vi "Physical Learning v2.vi"(4 "Learning Gains":dbl[](array[numeric])=[1.0, 1.0, 1.0, 0.0], 6 "PID Cluster":T4={"L1 to L4 PID Cluster"={"L1 PID Gains"={"Kp"=0.005, "Kd"=0.5, "Ki"=0.0005}, "L2 PID Gains"={"Kp"=0.01, "Kd"=1.0, "Ki"=0.005}, "L3 PID Gains"={"Kp"=0.05, "Kd"=1.0, "Ki"=0.0005}, "L4 PID Gains"={"Kp"=0.1, "Kd"=0.1, "Ki"=0.0005}}, "Stage PID Cluster"={"Stage Z PID"={"Kp"=0.0005, "Kd"=0.001, "Ki"=0.0}, "Stage Y PID"={"Kp"=0.0003, "Kd"=0.01, "Ki"=0.0}, "Stage X PID"={"Kp"=0.0003, "Kd"=0.01, "Ki"=0.0}}, "OCT Z PID Gains"={"Kp"=0.0003, "Kd"=0.0001, "Ki"=0.01}}, 7 "Input RUY":T5, 8 "error in":errorcluster, 9 "Offset Home 2 RCM":dbl[](array[numeric])=[0.0, 0.0, 0.0, 0.0], 10 "Prev Posit Cluster":T3={"Prev L1 to L4 Posit"=[-0.5319, -0.035669172703475985, -2.0566170657346783, 0.9099264705882353], "Prev Stage Posit"=[6.002553885707208, 5.996566124542428, 5.995469940427586], "Prev OCT Z Posit"=-0.0}, 11 "FPGA VI Reference In":refnum<k20>) -> (0 "error out":errorcluster, 1 "Updated Trajectory":T1, 2 "Last Posit Cluster":T2={"Last L1 to L4 Posit"=[0.0, 0.0, 0.0, 0.0], "Last Stage Posit"=[6.0, 6.0, 6.0], "Last OCT Z Posit"=0.0}, 3 "FPGA VI Reference Out":refnum<k20>, 5 "Updated RUY":T5)   [LabVIEW 2016]
uses:
  <vilib>/Platform/TimedLoop/XDataNode/timing_clust.ctl
  <vilib>/Platform/TimedLoop/XDataNode/nitl_modes.ctl
  <vilib>/Platform/TimedLoop/XDataNode/wakeup.ctl
  Global Variables.vi
  <vilib>/platform/TimedLoop/XDataNode/XDataNode.xnode
  <vilib>/Platform/TimedLoop/XDataNode/XDNodeRunTimeDep.lvlib
panel:
  out "In Servo Loop":bool
  out "Loading Finished":bool
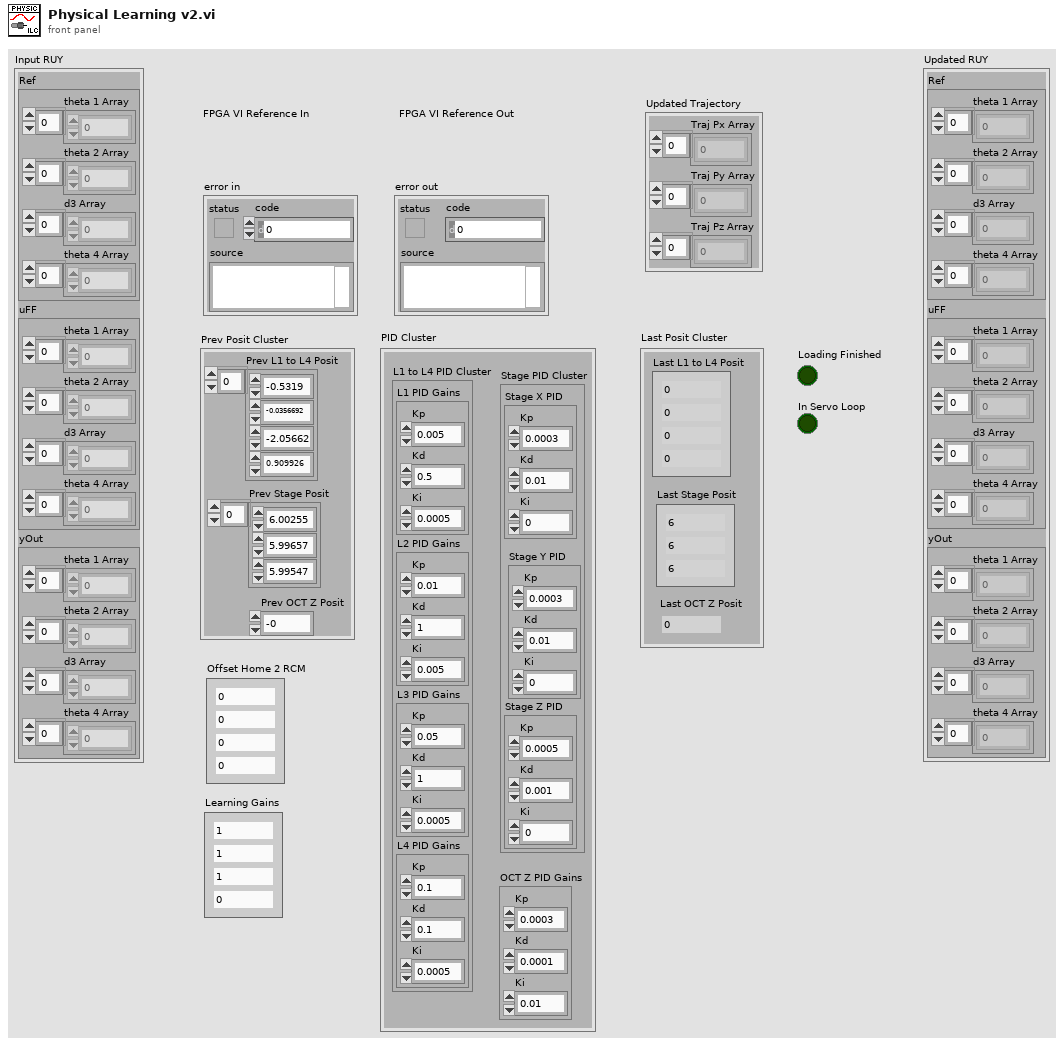
[diagram p1: front panel]
types:
  T1 = cluster{"Traj Px Array":dbl[], "Traj Py Array":dbl[], "Traj Pz Array":dbl[]}
  T2 = cluster{"Last L1 to L4 Posit":dbl[], "Last Stage Posit":dbl[], "Last OCT Z Posit":dbl}
  T3 = cluster{"Prev L1 to L4 Posit":dbl[], "Prev Stage Posit":dbl[], "Prev OCT Z Posit":dbl}
  T4 = cluster{"L1 to L4 PID Cluster":cluster{"L1 PID Gains":cluster{"Kp":dbl, "Kd":dbl, "Ki":dbl}, "L2 PID Gains":cluster{"Kp":dbl, "Kd":dbl, "Ki":dbl}, "L3 PID Gains":cluster{"Kp":dbl, "Kd":dbl, "Ki":dbl}, "L4 PID Gains":cluster{"Kp":dbl, "Kd":dbl, "Ki":dbl}}, "Stage PID Cluster":cluster{"Stage Z PID":cluster{"Kp":dbl, "Kd":dbl, "Ki":dbl}, "Stage Y PID":cluster{"Kp":dbl, "Kd":dbl, "Ki":dbl}, "Stage X PID":cluster{"Kp":dbl, "Kd":dbl, "Ki":dbl}}, "OCT Z PID Gains":cluster{"Kp":dbl, "Kd":dbl, "Ki":dbl}}
  T5 = cluster{"Ref":cluster{"theta 1 Array":dbl[], "theta 2 Array":dbl[], "d3 Array":dbl[], "theta 4 Array":dbl[]}, "uFF":cluster{"theta 1 Array":dbl[], "theta 2 Array":dbl[], "d3 Array":dbl[], "theta 4 Array":dbl[]}, "yOut":cluster{"theta 1 Array":dbl[], "theta 2 Array":dbl[], "d3 Array":dbl[], "theta 4 Array":dbl[]}}
  T6 = cluster{"Stop Vacuum":bool, "Vacuum Force":i8, "Max Limit [mmHg]":dbl, "Slide in":i8, "Irrigation?":bool}
  T7 = typedef "XDNodeRunTimeDep.lvlib/timing_clust.ctl" = cluster{"Expected End [f-1]":u64, "Actual End [f-1]":u64, "Finished Late? [f-1]":bool, "Expected End [i-1]":u64, "Actual End [i-1]":u64, "Finished Late? [i-1]":bool, "Expected Start [i]":u64, "Actual Start [i]":u64, "Expected Start [f]":u64, "Actual Start [f]":u64, "Source Name":string, "Structure Name":string, "Period":i64, "Deadline":i64, "Offset":i64, "Start":i64, "Priority":i32, "Timeout":i32, "Mode":T8, "Wakeup Reason":T9, "Error":errorcluster, "Source Type":string, "Secondary Source Type":string, "Global End Time":u64, "Global Start Time":u64, "Frame Duration":u64, "Iteration Duration":u64, "Assigned CPU":i32, "I/O Scan Engine Mode":u32}
  T8 = typedef "XDNodeRunTimeDep.lvlib/nitl_modes.ctl" = enum32{"No Change", "Process missed periods, maintain original phase", "Discard missed periods, maintain original phase", "Process missed periods, ignore original phase", "Discard missed periods, ignore original phase"}
  T9 = typedef "XDNodeRunTimeDep.lvlib/wakeup.ctl" = enum32{"Normal", "Aborted", "Asynchronous wakeup", "Timing source error", "Timed loop error", "Timeout"}
  T10 = cluster{"L1 PID Gains":cluster{"Kp":dbl, "Kd":dbl, "Ki":dbl}, "L2 PID Gains":cluster{"Kp":dbl, "Kd":dbl, "Ki":dbl}, "L3 PID Gains":cluster{"Kp":dbl, "Kd":dbl, "Ki":dbl}, "L4 PID Gains":cluster{"Kp":dbl, "Kd":dbl, "Ki":dbl}}
  T11 = cluster{"Stage Z PID":cluster{"Kp":dbl, "Kd":dbl, "Ki":dbl}, "Stage Y PID":cluster{"Kp":dbl, "Kd":dbl, "Ki":dbl}, "Stage X PID":cluster{"Kp":dbl, "Kd":dbl, "Ki":dbl}}
  T12 = cluster{"Accurus button":bool[], "Accurus engaged?":bool, "Vacuum Force":i32, "Accurus Ch. A Vout":dbl, "Accurus Ch. B Vout":dbl, "Irrigation engaged?":bool}
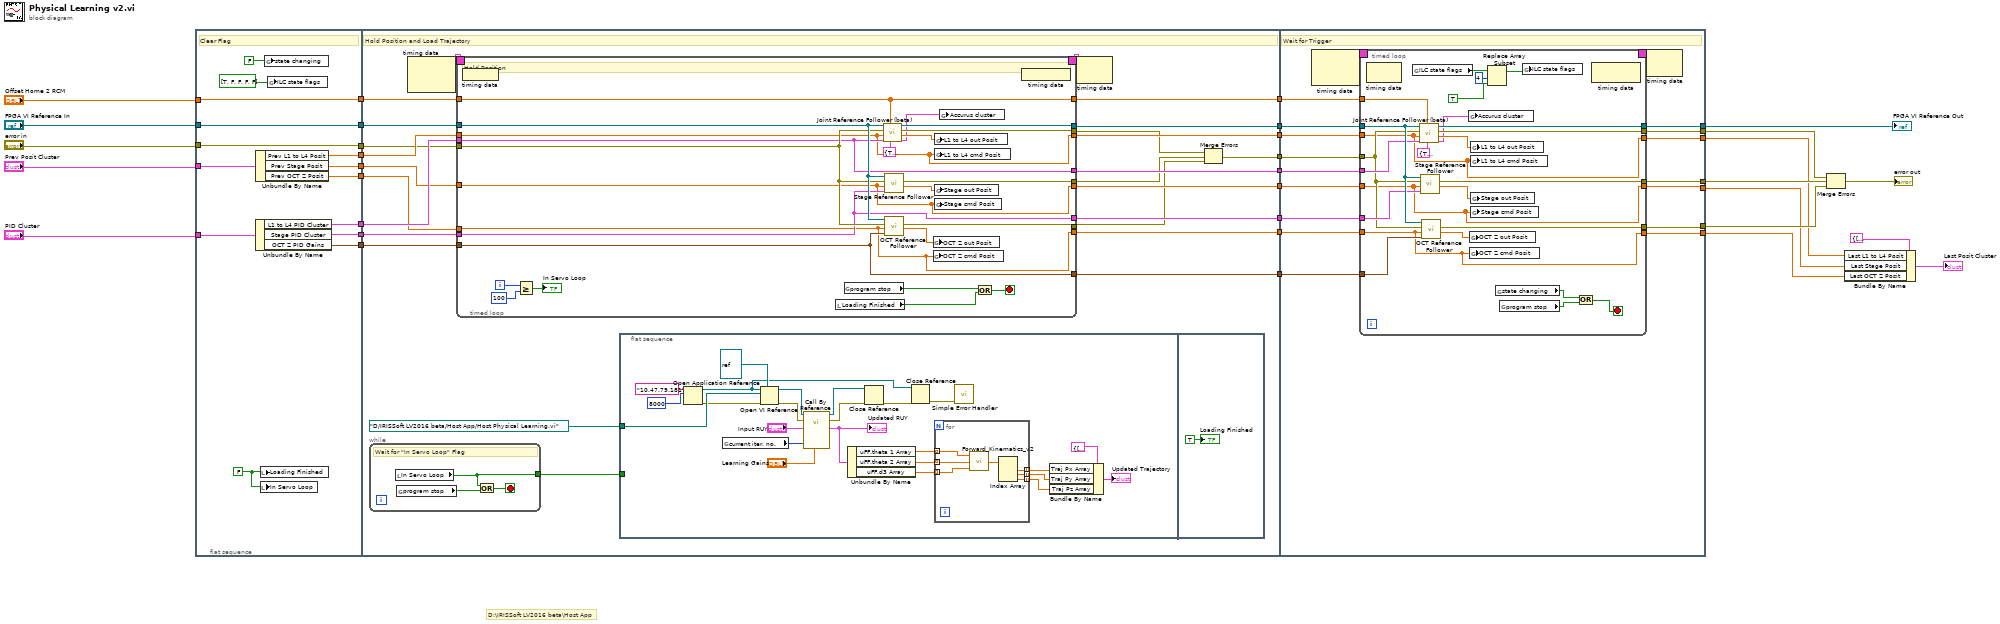
[diagram p0: block diagram]
diagram:
  # "D:\\IRISSoft LV2016 beta\\Host App"
  n1 = flat-sequence {
    tunnel: [w46] -> w33
    tunnel: "FPGA VI Reference In" -> [w46]
    tunnel: [w45] -> w32
    tunnel: "error in" -> [w45]
    tunnel: "Prev Posit Cluster" -> [w44]
    tunnel: "PID Cluster" -> [w43]
    tunnel: [w42] -> w31
    tunnel: [w41] -> w30
    tunnel: "Offset Home 2 RCM" -> [w40]
    tunnel: [w40] -> w29
    tunnel: [w39] -> w28
    tunnel: [w38] -> w27
    tunnel: [w37] -> w26
    tunnel: [w36] -> w25
    tunnel: w33 -> [w60]
    tunnel: w32 -> [w55]
    tunnel: w31 -> [w57]
    tunnel: w30 -> [w56]
    tunnel: w29 -> [w61]
    tunnel: w28 -> [w59]
    tunnel: w27 -> [w54]
    tunnel: w26 -> [w53]
    tunnel: w25 -> [w58]
    tunnel: [w72] -> w24
    tunnel: [w71] -> w23
    tunnel: [w70] -> w22
    tunnel: [w69] -> w21
    tunnel: [w68] -> w20
    tunnel: [w67] -> w19
    tunnel: [w66] -> w18
    tunnel: [w65] -> w17
    tunnel: [w49] -> w16
    tunnel: w24 -> [w151]
    tunnel: [w150] -> w9
    tunnel: [w149] -> w8
    tunnel: [w148] -> w7
    tunnel: w23 -> [w147]
    tunnel: w22 -> [w146]
    tunnel: w21 -> [w145]
    tunnel: w20 -> [w144]
    tunnel: w19 -> [w143]
    tunnel: w18 -> [w142]
    tunnel: w17 -> [w141]
    tunnel: [w140] -> w5
    tunnel: [w139] -> w4
    tunnel: [w138] -> w3
    tunnel: [w137] -> w1
    tunnel: w16 -> [w136]
    frame #0 {
      w35 = FALSE ("Loading Finished")
      # "Clear Flag"
      n2 = Unbundle By Name(w43) -> ("L1 to L4 PID Cluster"=w41:T10, "Stage PID Cluster"=w42:T11, "OCT Z PID Gains"=w36:cluster{"Kp":dbl, "Kd":dbl, "Ki":dbl})
      n3 = Unbundle By Name(w44) -> ("Prev L1 to L4 Posit"=w39:dbl[], "Prev Stage Posit"=w38:dbl[], "Prev OCT Z Posit"=w37:dbl)
      n4 = local write "Loading Finished"(w35) -> ()
      n5 = local write "In Servo Loop"(w35) -> ()
      n6 = global write "Global Variables.vi" "state changing"(FALSE ("state changing")) -> ()
      n7 = global write "Global Variables.vi" "ILC state flags"(bool[] [TRUE, FALSE, FALSE, FALSE, FALSE]) -> ()
    }
    frame #1 {
      # "Hold Position and Load Trajectory"
      n8 = while {
        tunnel: [w74] -> w62
        stop <- w75 stop-if-true
        # "Wait for \"In Servo Loop\" Flag"
        n9 = local read "In Servo Loop"() -> (w74:bool)
        n10 = global read "Global Variables.vi" "program stop"() -> (w73:bool)
        n11 = Or(x=w74, y=w73) -> (x .or. y?=w75:bool)
      }
      n12 = node-c288() -> (w64:T7)  [unwired: 2 in]
      n13 = timed-loop {
        timing: w64 -> [_]
        timing-out: [_] -> w63
        tunnel: w59 -> [w109]
        tunnel: w54 -> [w110]
        tunnel: w57 -> [w116]
        tunnel: w56 -> [w117]
        tunnel: w55 -> [w127]
        tunnel: w60 -> [w128]
        tunnel: w61 -> [w123]
        tunnel: w53 -> [w108]
        tunnel: w58 -> [w118]
        tunnel: [w109] -> w70
        tunnel: [w110] -> w69
        tunnel: [w108] -> w68
        tunnel: [w123] -> w71
        tunnel: [w122] -> w72
        tunnel: [w121] -> w52
        tunnel: [w120] -> w51
        tunnel: [w119] -> w50
        tunnel: [w118] -> w67
        tunnel: [w117] -> w66
        tunnel: [w116] -> w65
        i -> [w115]
        stop <- w131 stop-if-true
        # "Hold Position"
        n14 = node-c288 ("Output Node")() -> ()  [unwired: 1 in]
        n15 = Greater Or Equal?(x=w115, y=100) -> (x >= y?=→"In Servo Loop":bool)
        n16 = local read "Loading Finished"() -> (w130:bool)
        n17 = global read "Global Variables.vi" "program stop"() -> (w129:bool)
        n18 = call "Joint Reference Follower (beta).vi"("Accurus Ctrl Cluster"=T6 {"Stop Vacuum"=TRUE, "Vacuum Force"=0, "Max Limit [mmHg]"=600.0, "Slide in"=0, "Irrigation?"=TRUE}, "Offset Home2RCM [deg/mm]"=w123, "PID Ctrl Cluster"=w117, "Ref Array [deg/mm]"=w109, "error in"=w127, "FPGA VI Reference In"=w128) -> ("Accurus Output Cluster"=w111:T12, "Output Posit Array [deg/mm]"=w126:dbl[], "error out"=w121:errorcluster, "FPGA VI Reference Out"=w122:refnum<k20>)  [unwired: 2 in]
        n19 = call "Stage Reference Follower.vi"("Stage PID Cluster"=w116, "Stage cmd Posit [mm]"=w110, "error in"=w127, "FPGA VI Reference In"=w128) -> ("Stage out Posit [mm]"=w125:dbl[], "error out"=w120:errorcluster)  [unwired: 5 in, 1 out]
        n20 = call "OCT Reference Follower.vi"("OCT Z PID Gains"=w118, "OCT  Z cmd Posit [mm]"=w108, "error in"=w127, "FPGA VI Reference In"=w128) -> ("OCT  Z out Posit [mm]"=w124:dbl, "error out"=w119:errorcluster)  [unwired: 5 in, 1 out]
        n21 = global write "Global Variables.vi" "OCT Z out Posit"(w124) -> ()
        n22 = global write "Global Variables.vi" "OCT Z cmd Posit"(w108) -> ()
        n23 = global write "Global Variables.vi" "L1 to L4 out Posit"(w126) -> ()
        n24 = global write "Global Variables.vi" "L1 to L4 cmd Posit"(w109) -> ()
        n25 = global write "Global Variables.vi" "Stage out Posit"(w125) -> ()
        n26 = global write "Global Variables.vi" "Stage cmd Posit"(w110) -> ()
        n27 = global write "Global Variables.vi" "Accurus cluster"(w111) -> ()
        n28 = Or(x=w129, y=w130) -> (x .or. y?=w131:bool)
        n29 = node-c288() -> ()  [unwired: 1 out]
      }
      n30 = flat-sequence {
        tunnel: w62 -> [_]
        tunnel: path "D:/IRISSoft LV2016 beta/Host App/Host Physical Learning.vi" ("vi path") -> [w91]
        frame #0 {
          n31 = Open Application Reference(10:u16 8000 ("port number or service name (3363)"), 11:"10.47.79.181" ("machine name (\"\":  open local reference)")) -> (0:w88:errorcluster, 3:w93:refnum<vi>)  [unwired: 2 in]
          n32 = global read "Global Variables.vi" "current iter. no."() -> (w86:u16)
          n33 = Open VI Reference(type specifier VI Refnum (for type only)=refnum<vi> refnum, application reference (local)=w93, vi path=w91, error in (no error)=w88) -> (vi reference=w95:refnum<vi>, error out=w90:errorcluster)  [unwired: 2 in]
          n34 = call-by-ref "?"(reference=w95, error in=w90, "Learning Gains"="Learning Gains", "Curr Iter No"=w86, "Input RUY"="Input RUY") -> (reference out=w96:refnum<vi>, error out=w89:errorcluster, "Updated RUY"=w84:T5)  [unwired: 8 in]
          "Updated RUY" <- w84
          n35 = Unbundle By Name(w84) -> ("uFF.theta 1 Array"=w82:dbl[], "uFF.theta 2 Array"=w81:dbl[], "uFF.d3 Array"=w80:dbl[])
          n36 = Close Reference(reference=w96, error in (no error)=w89) -> (error out=w92:errorcluster)
          n37 = Close Reference(reference=w93, error in (no error)=w92) -> (error out=w87:errorcluster)
          n38 = for {
            tunnel: w82 -> [w106] mode=indexing
            tunnel: w81 -> [w105] mode=indexing
            tunnel: w80 -> [w104] mode=indexing
            tunnel: [w102] -> w79 mode=indexing
            tunnel: [w101] -> w78 mode=indexing
            tunnel: [w100] -> w77 mode=indexing
            n39 = call "Forward_Kinematics_v2.vi"("theta 3"=w104, "theta 2"=w105, "theta 1"=w106) -> ("position"=w103:dbl[])
            n40 = Index Array(array=w103) -> (element #1=w102:dbl, element #2=w101:dbl, element #3=w100:dbl)  [unwired: 3 in]
          }
          n41 = call <vilib>:"Simple Error Handler.vi"("error in (no error)"=w87) -> ()  [unwired: 4 in, 5 out]
          n42 = Bundle By Name(cluster=T1 {"Traj Px Array"=[], "Traj Py Array"=[], "Traj Pz Array"=[]} ("Trajectory Cluster"), "Traj Px Array"=w79, "Traj Py Array"=w78, "Traj Pz Array"=w77) -> (→"Updated Trajectory":T1)
        }
        frame #1 {
          "Loading Finished" <- TRUE ("Loading Finished")
        }
      }
      n43 = node-c288(w63) -> ()  [unwired: 1 out]
      n44 = Merge Errors(w52, w51, w50) -> (w49:errorcluster)
    }
    frame #2 {
      # "Wait for Trigger"
      n45 = node-c288() -> (w153:T7)  [unwired: 2 in]
      n46 = timed-loop {
        timing: w153 -> [_]
        timing-out: [_] -> w152
        tunnel: w151 -> [w171]
        tunnel: [w170] -> w149
        tunnel: [w169] -> w150
        tunnel: [w168] -> w148
        tunnel: w147 -> [w167]
        tunnel: w146 -> [w156]
        tunnel: w145 -> [w155]
        tunnel: w144 -> [w154]
        tunnel: w143 -> [w166]
        tunnel: w142 -> [w165]
        tunnel: w141 -> [w164]
        tunnel: [w156] -> w140
        tunnel: [w155] -> w139
        tunnel: [w154] -> w138
        tunnel: [w160] -> w137
        tunnel: w136 -> [w159]
        stop <- w178 stop-if-true
        n47 = node-c288() -> ()  [unwired: 1 in, 1 out]
        n48 = global read "Global Variables.vi" "ILC state flags"() -> (w175:bool[])
        n49 = call "Joint Reference Follower (beta).vi"("Accurus Ctrl Cluster"=T6 {"Stop Vacuum"=TRUE, "Vacuum Force"=0, "Max Limit [mmHg]"=600.0, "Slide in"=0, "Irrigation?"=TRUE}, "Offset Home2RCM [deg/mm]"=w167, "PID Ctrl Cluster"=w165, "Ref Array [deg/mm]"=w156, "error in"=w159, "FPGA VI Reference In"=w171) -> ("Accurus Output Cluster"=w157:T12, "Output Posit Array [deg/mm]"=w163:dbl[], "error out"=w170:errorcluster, "FPGA VI Reference Out"=w160:refnum<k20>)  [unwired: 2 in]
        n50 = call "Stage Reference Follower.vi"("Stage PID Cluster"=w164, "Stage cmd Posit [mm]"=w155, "error in"=w159, "FPGA VI Reference In"=w171) -> ("Stage out Posit [mm]"=w162:dbl[], "error out"=w169:errorcluster)  [unwired: 5 in, 1 out]
        n51 = call "OCT Reference Follower.vi"("OCT Z PID Gains"=w166, "OCT  Z cmd Posit [mm]"=w154, "error in"=w159, "FPGA VI Reference In"=w171) -> ("OCT  Z out Posit [mm]"=w161:dbl, "error out"=w168:errorcluster)  [unwired: 5 in, 1 out]
        n52 = global write "Global Variables.vi" "Accurus cluster"(w157) -> ()
        n53 = global write "Global Variables.vi" "OCT Z out Posit"(w161) -> ()
        n54 = global write "Global Variables.vi" "OCT Z cmd Posit"(w154) -> ()
        n55 = global write "Global Variables.vi" "L1 to L4 out Posit"(w163) -> ()
        n56 = global write "Global Variables.vi" "L1 to L4 cmd Posit"(w156) -> ()
        n57 = global write "Global Variables.vi" "Stage out Posit"(w162) -> ()
        n58 = global write "Global Variables.vi" "Stage cmd Posit"(w155) -> ()
        n59 = Replace Array Subset(array=w175, new element=TRUE ("new element/subarray"), index=4) -> (w174:bool[])
        n60 = global read "Global Variables.vi" "state changing"() -> (w177:bool)
        n61 = global read "Global Variables.vi" "program stop"() -> (w176:bool)
        n62 = global write "Global Variables.vi" "ILC state flags"(w174) -> ()
        n63 = Or(x=w177, y=w176) -> (x .or. y?=w178:bool)
        n64 = node-c288() -> ()  [unwired: 1 in, 1 out]
      }
      n65 = node-c288(w152) -> ()  [unwired: 1 out]
    }
  }
  n66 = Merge Errors(w8, w9, w7) -> (→"error out":errorcluster)
  n67 = Bundle By Name(cluster=T2 {"Last L1 to L4 Posit"=[0.0, 0.0, 0.0, 0.0], "Last Stage Posit"=[6.0, 6.0, 6.0], "Last OCT Z Posit"=0.0} ("Last Posit Cluster 2"), "Last L1 to L4 Posit"=w5, "Last Stage Posit"=w4, "Last OCT Z Posit"=w3) -> (→"Last Posit Cluster":T2)
  "FPGA VI Reference Out" <- w1
